vi "Scale.vi"(8 "error in (no error)":errorcluster, 10 "Scale Factor":dbl, 11 "Rectangle in":refnum<class "Rectangle.lvclass">) -> (0 "error out":errorcluster, 3 "Rectangle out":refnum<class "Rectangle.lvclass">)   [LabVIEW 2021, in "Picture2D.lvlib" / "Rectangle.lvclass"]
uses:
  Rectangle.lvclass
  Rectangle.lvclass/Rectangle.ctl
  Polygone/Polygone.lvclass
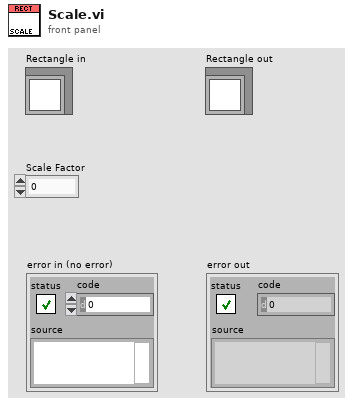
[diagram p1: front panel]
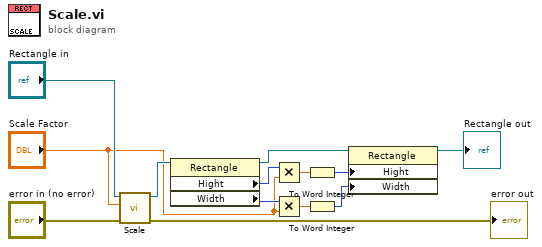
[diagram p0: block diagram]
diagram:
  n1 = call-parent "Scale.vi"("error in (no error)"="error in (no error)", "Scale Factor"="Scale Factor", "Shape in"="Rectangle in") -> ("error out"=→"error out":errorcluster, "Shape out"=w10:refnum<class "Rectangle.lvclass">)  [unwired: 7 in]
  n2 = property class="Rectangle"(reference=w10) -> (reference out=w1:refnum<class "Rectangle.lvclass">, "Hight"=w9:i16, "Width"=w8:i16)  [unwired: 1 in, 1 out]
  n3 = Multiply(x=w9, y="Scale Factor") -> (x*y=w5:dbl)
  n4 = Multiply(x=w8, y="Scale Factor") -> (x*y=w6:dbl)
  n5 = To Word Integer(number=w5) -> (16bit integer=w3:i16)
  n6 = To Word Integer(number=w6) -> (16bit integer=w4:i16)
  n7 = property class="Rectangle"(reference=w1, "Hight"=w3, "Width"=w4) -> (reference out=→"Rectangle out":refnum<class "Rectangle.lvclass">)  [unwired: 1 in, 1 out]
